vi "Update Size Limits.vi"(0 "Guest Manager UI in":refnum<class "Guest Manager UI.lvclass">, 5 "Adult Count":u32, 7 "Children Count":u32, 11 "error in (no error)":errorcluster) -> (4 "Guest Manager UI out":refnum<class "Guest Manager UI.lvclass">, 15 "error out":errorcluster)   [LabVIEW 2023, in "Guest Manager UI.lvlib" / "Guest Manager UI.lvclass"]
uses:
  Guest Manager UI.lvclass
  Guest Manager UI.lvclass/Guest Manager UI.ctl
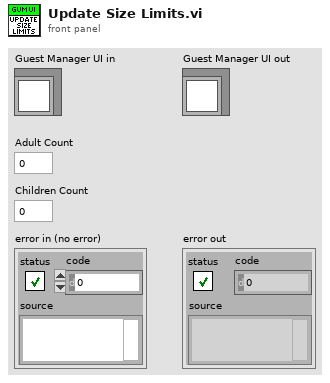
[diagram p1: front panel]
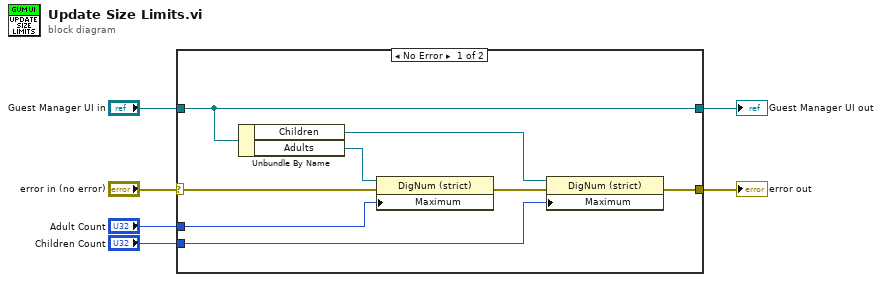
[diagram p0: block diagram]
diagram:
  n1 = case shown="No Error" "error in (no error)" {
    selector: "error in (no error)" -> [w14 w16]
    tunnel: [w8 w16] -> w5
    tunnel: [w13 w15] -> w3
    tunnel: "Guest Manager UI in" -> [w13 w15]
    tunnel: "Adult Count" -> [w11 _]
    tunnel: "Children Count" -> [w7 _]
    frame No Error {
      n2 = Unbundle By Name(w13) -> ("Children"=w9:refnum<vi>, "Adults"=w12:refnum<vi>)
      n3 = property class="DigNum (strict)"(reference=w12, error in=w14, "Maximum"=w11) -> (error out=w10:errorcluster)  [unwired: 1 out]
      n4 = property class="DigNum (strict)"(reference=w9, error in=w10, "Maximum"=w7) -> (error out=w8:errorcluster)  [unwired: 1 out]
    }
    frame Error {
    }
  }
  "error out" <- w5
  "Guest Manager UI out" <- w3
